vi "Sim Spectrum Capture.vi"(10 "Wavelength Axis":i32[](array[numeric]), 11 "Time Point":dbl) -> (2 "Captured Spectrum Out":dbl[](array[numeric]))   [LabVIEW 2010]
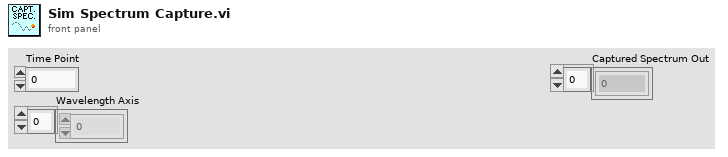
[diagram p1: front panel]
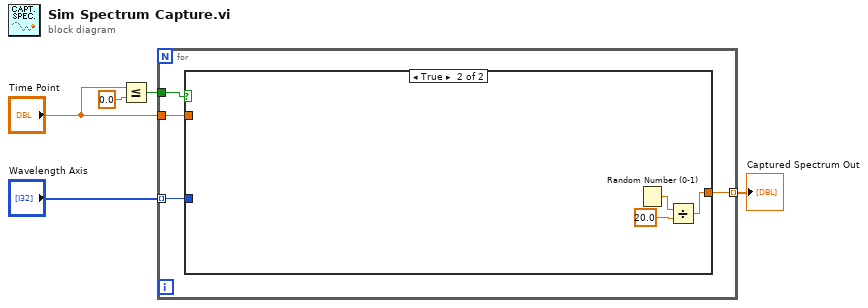
[diagram p0: block diagram]
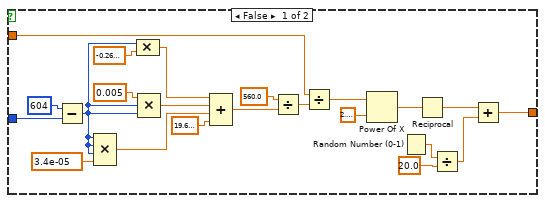
[diagram p2: hidden frame]
diagram:
  n1 = Less Or Equal?(x="Time Point", y=0.0) -> (x <= y?=w4:bool)
  n2 = for {
    tunnel: "Wavelength Axis" -> [w6] mode=indexing
    tunnel: w4 -> [w9]
    tunnel: "Time Point" -> [w8]
    tunnel: [w7] -> w1 mode=indexing
    n3 = case shown="True" w9 {
      tunnel: w8 -> [w30 _]
      tunnel: [w14 w33] -> w7
      tunnel: w6 -> [w17 _]
      frame False {
        n4 = Subtract(x=604 ("x 2"), y=w17) -> (x-y=w16:i32)
        n5 = Compound Arithmetic op=MULTIPLY(w16, w16, w16, 3.4e-05 ("a")) -> (w22:dbl)
        n6 = Compound Arithmetic op=MULTIPLY(w16, -0.26000000000000006 ("c")) -> (w24:dbl)
        n7 = Compound Arithmetic op=MULTIPLY(0.005 ("b"), w16, w16) -> (w23:dbl)
        n8 = Compound Arithmetic op=ADD(w24, w23, w22, 19.60000000000001 ("d")) -> (w18:dbl)
        n9 = Divide(x=560.0, y=w18) -> (x/y=w20:dbl)
        n10 = Divide(x=w30, y=w20) -> (x/y=w28:dbl)
        n11 = Power Of X(1:2.718281828459045, 2:w28) -> (0:w29:dbl)
        n12 = Random Number (0-1)() -> (number: 0 to 1=w12:dbl)
        n13 = Reciprocal(x=w29) -> (1/x=w13:dbl)
        n14 = Divide(x=w12, y=20.0) -> (x/y=w11:dbl)
        n15 = Add(x=w13, y=w11) -> (x+y=w14:dbl)
      }
      frame True {
        n16 = Random Number (0-1)() -> (number: 0 to 1=w34:dbl)
        n17 = Divide(x=w34, y=20.0) -> (x/y=w33:dbl)
      }
    }
  }
  "Captured Spectrum Out" <- w1
